vi "smith_analysis.vi"() -> ()   [LabVIEW 2013]
panel:
  out "appended array":dbl[][](array[numeric])=[[9086390000.0, 9086990000.0, 9087590000.0, 9088190000.0, 9088790000.0, 9089390000.0, 9089990000.0, 9090590000.0, 9091190000.0, 9091790000.0, 9092390000.0, 9092990000.0, 9093590000.0, 9094190000.0, 9094790000.0, 9095390000.0, 9095990000.0, 9096590000.0, 9097190000.0, 9097790000.0, 9098390000.0, 9098990000.0, 9099590000.0, 9100190000.0, 9100790000.0, 9101390000.0, 9101990000.0, 9102590000.0, 9103190000.0, 9103790000.0, 9104390000.0, 9104990000.0, 9105590000.0, 9106190000.0, 9106790000.0, 9107390000.0, 9107990000.0, 9108590000.0, 9109190000.0, 9109790000.0, 9110390000.0, 9110990000.0, 9111590000.0, 9112190000.0, 9112790000.0, 9113390000.0, 9113990000.0, 9114590000.0, 9115190000.0, 9115790000.0, 9116390000.0, 9116990000.0, 9117590000.0, 9118190000.0, 9118790000.0, 9119390000.0, 9119990000.0, 9120590000.0, 9121190000.0, 9121790000.0, 9122390000.0, 9122990000.0, 9123590000.0, 9124190000.0, 9124790000.0, 9125390000.0, 9125990000.0, 9126590000.0, 9127190000.0, 9127790000.0, 9128390000.0, 9128990000.0, 9129590000.0, 9130190000.0, 9130790000.0, 9131390000.0, 9131990000.0, 9132590000.0, 9133190000.0, 9133790000.0, 9134390000.0, 9134990000.0, 9135590000.0, 9136190000.0, 9136790000.0, 9137390000.0, 9137990000.0, 9138590000.0, 9139190000.0, 9139790000.0, 9140390000.0, 9140990000.0, 9141590000.0, 9142190000.0, 9142790000.0, 9143390000.0, 9143990000.0, 9144590000.0, 9145190000.0, 9145790000.0, 9146390000.0, 9146990000.0, 9147590000.0, 9148190000.0, 9148790000.0, 9149390000.0, 9149990000.0, 9150590000.0, 9151190000.0, 9151790000.0, 9152390000.0, 9152990000.0, 9153590000.0, 9154190000.0, 9154790000.0, 9155390000.0, 9155990000.0, 9156590000.0, 9157190000.0, 9157790000.0, 9158390000.0, 9158990000.0, 9159590000.0, 9160190000.0, 9160790000.0, 9161390000.0, 9161990000.0, 9162590000.0, 9163190000.0, 9163790000.0, 9164390000.0, 9164990000.0, 9165590000.0, 9166190000.0, 9166790000.0, 9167390000.0, 9167990000.0, 9168590000.0, 9169190000.0, 9169790000.0, 9170390000.0, 9170990000.0, 9171590000.0, 9172190000.0, 9172790000.0, 9173390000.0, 9173990000.0, 9174590000.0, 9175190000.0, 9175790000.0, 9176390000.0, 9176990000.0, 9177590000.0, 9178190000.0, 9178790000.0, 9179390000.0, 9179990000.0, 9180590000.0, 9181190000.0, 9181790000.0, 9182390000.0, 9182990000.0, 9183590000.0, 9184190000.0, 9184790000.0, 9185390000.0, 9185990000.0, 9186590000.0, 9187190000.0, 9187790000.0, 9188390000.0, 9188990000.0, 9189590000.0, 9190190000.0, 9190790000.0, 9191390000.0, 9191990000.0, 9192590000.0, 9193190000.0, 9193790000.0, 9194390000.0, 9194990000.0, 9195590000.0, 9196190000.0, 9196790000.0, 9197390000.0, 9197990000.0, 9198590000.0, 9199190000.0, 9199790000.0, 9200390000.0, 9200990000.0, 9201590000.0, 9202190000.0, 9202790000.0, 9203390000.0, 9203990000.0, 9204590000.0, 9205190000.0, 9205790000.0, 9206390000.0, 9206990000.0, 9207590000.0, 9208190000.0, 9208790000.0, 9209390000.0, 9209990000.0, 9210590000.0, 9211190000.0, 9211790000.0, 9212390000.0, 9212990000.0, 9213590000.0, 9214190000.0, 9214790000.0, 9215390000.0, 9215990000.0, 9216590000.0, 9217190000.0, 9217790000.0, 9218390000.0, 9218990000.0, 9219590000.0, 9220190000.0, 9220790000.0, 9221390000.0, 9221990000.0, 9222590000.0, 9223190000.0, 9223790000.0, 9224390000.0, 9224990000.0, 9225590000.0, 9226190000.0, 9226790000.0, 9227390000.0, 9227990000.0, 9228590000.0, 9229190000.0, 9229790000.0, 9230390000.0, 9230990000.0, 9231590000.0, 9232190000.0, 9232790000.0, 9233390000.0, 9233990000.0, 9234590000.0, 9235190000.0, 9235790000.0, 9236390000.0, 9236990000.0, 9237590000.0, 9238190000.0, 9238790000.0, 9239390000.0, 9239990000.0, 9240590000.0, 9241190000.0, 9241790000.0, 9242390000.0, 9242990000.0, 9243590000.0, 9244190000.0, 9244790000.0, 9245390000.0, 9245990000.0, 9246590000.0, 9247190000.0, 9247790000.0, 9248390000.0, 9248990000.0, 9249590000.0, 9250190000.0, 9250790000.0, 9251390000.0, 9251990000.0, 9252590000.0, 9253190000.0, 9253790000.0, 9254390000.0, 9254990000.0, 9255590000.0, 9256190000.0, 9256790000.0, 9257390000.0, 9257990000.0, 9258590000.0, 9259190000.0, 9259790000.0, 9260390000.0, 9260990000.0, 9261590000.0, 9262190000.0, 9262790000.0, 9263390000.0, 9263990000.0, 9264590000.0, 9265190000.0, 9265790000.0, 9266390000.0, 9266990000.0, 9267590000.0, 9268190000.0, 9268790000.0, 9269390000.0, 9269990000.0, 9270590000.0, 9271190000.0, 9271790000.0, 9272390000.0, 9272990000.0, 9273590000.0, 9274190000.0, 9274790000.0, 9275390000.0, 9275990000.0, 9276590000.0, 9277190000.0, 9277790000.0, 9278390000.0, 9278990000.0, 9279590000.0, 9280190000.0, 9280790000.0, 9281390000.0, 9281990000.0, 9282590000.0, 9283190000.0, 9283790000.0, 9284390000.0, 9284990000.0, 9285590000.0, 9286190000.0, 9286790000.0, 9287390000.0, 9287990000.0, 9288590000.0, 9289190000.0, 9289790000.0, 9290390000.0, 9290990000.0, 9291590000.0, 9292190000.0, 9292790000.0, 9293390000.0, 9293990000.0, 9294590000.0, 9295190000.0, 9295790000.0, 9296390000.0, 9296990000.0, 9297590000.0, 9298190000.0, 9298790000.0, 9299390000.0, 9299990000.0, 9300590000.0, 9301190000.0, 9301790000.0, 9302390000.0, 9302990000.0, 9303590000.0, 9304190000.0, 9304790000.0, 9305390000.0, 9305990000.0, 9306590000.0, 9307190000.0, 9307790000.0, 9308390000.0, 9308990000.0, 9309590000.0, 9310190000.0, 9310790000.0, 9311390000.0, 9311990000.0, 9312590000.0, 9313190000.0, 9313790000.0, 9314390000.0, 9314990000.0, 9315590000.0, 9316190000.0, 9316790000.0, 9317390000.0, 9317990000.0, 9318590000.0, 9319190000.0, 9319790000.0, 9320390000.0, 9320990000.0, 9321590000.0, 9322190000.0, 9322790000.0, 9323390000.0, 9323990000.0, 9324590000.0, 9325190000.0, 9325790000.0, 9326390000.0, 9326990000.0, 9327590000.0, 9328190000.0, 9328790000.0, 9329390000.0, 9329990000.0, 9330590000.0, 9331190000.0, 9331790000.0, 9332390000.0, 9332990000.0, 9333590000.0, 9334190000.0, 9334790000.0, 9335390000.0, 9335990000.0, 9336590000.0, 9337190000.0, 9337790000.0, 9338390000.0, 9338990000.0, 9339590000.0, 9340190000.0, 9340790000.0, 9341390000.0, 9341990000.0, 9342590000.0, 9343190000.0, 9343790000.0, 9344390000.0, 9344990000.0, 9345590000.0, 9346190000.0, 9346790000.0, 9347390000.0, 9347990000.0, 9348590000.0, 9349190000.0, 9349790000.0, 9350390000.0, 9350990000.0, 9351590000.0, 9352190000.0, 9352790000.0, 9353390000.0, 9353990000.0, 9354590000.0, 9355190000.0, 9355790000.0, 9356390000.0, 9356990000.0, 9357590000.0, 9358190000.0, 9358790000.0, 9359390000.0, 9359990000.0, 9360590000.0, 9361190000.0, 9361790000.0, 9362390000.0, 9362990000.0, 9363590000.0, 9364190000.0, 9364790000.0, 9365390000.0, 9365990000.0, 9366590000.0, 9367190000.0, 9367790000.0, 9368390000.0, 9368990000.0, 9369590000.0, 9370190000.0, 9370790000.0, 9371390000.0, 9371990000.0, 9372590000.0, 9373190000.0, 9373790000.0, 9374390000.0, 9374990000.0, 9375590000.0, 9376190000.0, 9376790000.0, 9377390000.0, 9377990000.0, 9378590000.0, 9379190000.0, 9379790000.0, 9380390000.0, 9380990000.0, 9381590000.0, 9382190000.0, 9382790000.0, 9383390000.0, 9383990000.0, 9384590000.0, 9385190000.0, 9385790000.0, 0.0], [1.0014470756472609, 0.9811749599727149, 0.975937039152533, 0.957404308515006, 0.9736018230093859, 0.9604604054761811, 0.9792049244201155, 1.0152541903970067, 1.004440422987172, 0.9669142300691471, 0.9778889586067279, 0.9827563524115415, 0.9889865842957853, 0.9705799067333685, 1.0100148361341221, 0.9773606743960654, 0.9646774483545443, 0.9704643155585843, 0.9783010544752769, 0.9951174837276988, 0.9574011288539037, 0.9859926147182249, 0.9669596436669335, 0.9920583106963926, 0.9854864109639495, 0.9799430549111374, 0.9769108482599617, 1.034057942667083, 0.9639858725088492, 0.9893429207880235, 0.9909416773256717, 0.9890686668064436, 0.983690008455327, 0.992837107143869, 0.9537054075489657, 1.0007092044221306, 0.9859170574219019, 0.9924581976110967, 0.9633179253367699, 0.9854993598276752, 0.9988614892860668, 1.004290542828067, 0.9951406919895751, 0.9595604473467628, 0.9755040689387509, 1.0066850706289576, 0.9666753740843728, 0.9797492943616066, 0.9891009789576483, 0.976218574351781, 0.9423483466974647, 0.9949809297127765, 0.9863441817937338, 0.9948322048119537, 0.981473364768583, 0.9999575553906259, 0.9933478773682365, 0.9952508245668754, 0.9823564820622492, 0.9847369655634216, 1.0210893363673963, 0.9954525985294357, 1.0004858497317275, 0.9660627936505503, 0.9850142439017647, 0.9689016818726742, 0.9772122398202737, 0.9773991677095369, 0.995057165612707, 0.9794999128822224, 0.9653556017088364, 0.9590793894023546, 0.9927546646176238, 0.973951113405735, 0.998351636736338, 0.97956788821144, 0.9539799170177218, 0.9835730149003353, 0.9872478691492744, 1.0022504649650081, 0.9943597265449575, 1.007315613095887, 1.016783886043785, 0.9699349529618666, 1.0102763892837336, 0.9819198699224674, 1.0011398706228367, 0.9854156883054559, 1.0057695829277393, 0.9742808082199741, 0.983537484305779, 0.9756139402394592, 0.9529997175528215, 0.9882672606378323, 0.9964646576378824, 1.0162769185869391, 0.9771113467798679, 0.9902362691931147, 0.9974945712236141, 0.9857676635027528, 0.990436808833684, 1.0100054750913074, 1.02277349272177, 0.9912131451821969, 0.9706813850121981, 0.9941292664957707, 0.9971653637847144, 0.9727308351939552, 0.9985557171670739, 0.990099281613391, 0.9592058080706113, 0.9850771730276339, 0.9579121848414565, 1.0413373602481122, 0.985479131778255, 0.9745571754831918, 0.9822577587259966, 1.0045577810317978, 0.9893107663949505, 0.979052992956135, 0.995395289845648, 1.003559463689938, 0.9627423299378147, 0.9818148736996156, 0.9911217507502924, 0.9691634713250117, 0.989465289500339, 0.9869127245666133, 1.0003808783369692, 0.9929945051626885, 1.0352322704115924, 0.9850581097960746, 0.9637516282967002, 0.9694897298412518, 0.9884441528397356, 0.995682923689632, 1.0029582140150322, 0.9816802190570769, 0.973562814550217, 0.9786970085879368, 1.0077631757583416, 0.9912918509414795, 0.9988234438690078, 0.9614578884461156, 0.9718322743908004, 0.9995513798844637, 1.0082429778200743, 1.0017536975084038, 1.0064115760126986, 0.9876507461851545, 0.956689385504372, 0.9661731716427335, 0.977175002325847, 0.9874001417065671, 0.9913195667202573, 1.0229947902987884, 0.9908230523450857, 0.9723595088037424, 1.0167086713851914, 1.0014221968876416, 0.9673383399753221, 0.9734357709886645, 0.9739288695081485, 0.9823171957631014, 0.9790041819946486, 0.9892116556181274, 0.9772477925686469, 1.0181758365556028, 1.001727376833795, 0.9683302069118086, 1.00198525147198, 0.9513182110513856, 0.9925278473984726, 0.9951607813898269, 0.9702746420708325, 0.9668003661435942, 0.9903244718945475, 1.0002563330224825, 0.9559761300224189, 0.974546529993097, 0.9995297116612798, 1.0046846903417743, 0.983485793116926, 1.0026831282008672, 0.9905199996322401, 0.9782269645034511, 1.0019674827158171, 0.9838323020512393, 0.9871369498901948, 1.0155032878430428, 1.0007802083671549, 0.9717739819680403, 0.9798965419234907, 0.9712219261120401, 0.9844985597447395, 0.9798576441835376, 0.9498016858038393, 0.9485857892398264, 0.9454073623982583, 1.0007271949801384, 0.9662435353148254, 0.9887495046962643, 0.9839744349092254, 0.9364946992801554, 0.9643564952803784, 0.9441374655249337, 0.971754009009434, 0.94475767751919, 0.9485826443001484, 0.9830282794482469, 0.9400594878438806, 0.9409738189508776, 0.9066711079610856, 0.915463647678557, 0.9396701651566188, 0.9520975581728508, 0.9423126541573191, 0.916329282360555, 0.921566191380927, 0.865778549512083, 0.8830002295417998, 0.9015180477343065, 0.8545954691171324, 0.8523334136356121, 0.8719727628977598, 0.8621363153292432, 0.8582191014270931, 0.8574731836182887, 0.8352852285636092, 0.8332663424689872, 0.8367676949759798, 0.8148731930380775, 0.768132593782985, 0.7554392738920802, 0.7742973748751909, 0.7692309771947555, 0.7361853856775491, 0.7229295395020657, 0.7162292618691556, 0.7153223511486996, 0.7038523932203432, 0.7046631520252984, 0.6876654171667271, 0.7131742885932114, 0.7295949009378736, 0.7202100019940961, 0.7169640294889787, 0.7255956374699953, 0.7200600365926345, 0.7328738917670794, 0.7451463019083417, 0.7501408073253467, 0.7860280564814197, 0.7502657987696241, 0.7949357397204114, 0.7308381467377276, 0.7339839462608265, 0.7818278743775611, 0.8228176839920871, 0.824930294322964, 0.7964975850050977, 0.851040653852145, 0.8674023224409153, 0.8329611929525236, 0.8653112375468961, 0.903797950771074, 0.904626553567601, 0.8942137089930287, 0.8929279570420267, 0.9161286665966389, 0.9213518446365686, 0.9337311542863986, 0.9132314115538239, 0.958929531207723, 0.9520449589749719, 0.9606968484432504, 0.9622764460410423, 0.9405015634503353, 0.9181830082029172, 0.9313713628937752, 0.9682831802106964, 0.9726380480876876, 0.9675825582307597, 0.9755855251096048, 0.9742205285306306, 0.938117519638244, 0.9894213001906471, 0.9623345999767065, 0.9579679485061534, 0.9742754606715178, 0.965359029778444, 0.9674215131103316, 0.999048768474733, 0.9660126446852795, 0.9718607497332871, 0.9884785831389925, 0.9889770052018733, 0.975942799652276, 0.9674709559003105, 0.9645214138379589, 0.9826473208551918, 0.9747900514559639, 1.0073417463170438, 0.9960191326890215, 0.9777628016062563, 0.9871572804153868, 0.979732602581617, 0.9621783501900804, 1.0035494562281797, 1.0234667718707915, 0.9744321465519066, 0.984978719422053, 0.9490304588181648, 0.960471232634771, 0.9586820282041454, 0.9952703809974975, 0.9935939138388714, 0.9798335301757216, 0.9818843448512631, 0.9981926711538844, 0.9667940944562141, 0.9930083650297539, 1.0042728940444805, 0.9833369795347292, 1.0017517424062143, 0.9753024253139055, 0.965200808574049, 0.9992128024341174, 0.9793024932726984, 1.0380638317887279, 1.00837436589276, 1.0087785666684708, 0.9932289237477132, 0.9881491713540708, 0.9823661949193174, 1.0071428430282414, 1.0047494405176227, 0.9697388231654123, 0.9955648663035147, 0.9757451117672439, 0.965899932555795, 0.995173946728936, 0.9733206750405338, 1.0100840183077469, 1.0205798795098242, 0.980784238323221, 0.9938809875634443, 0.9897960417826223, 0.9676963048194741, 0.9840107326075767, 0.9780538666413968, 0.989345322004715, 0.9725800113897322, 0.9962779298768482, 0.9932182218277528, 0.999048368598765, 0.997704205203082, 1.023055966550519, 0.9983091962952612, 1.0033860925619922, 1.001080262818101, 1.006336077516865, 0.9812156487589327, 0.9866191288790616, 0.9932778035890981, 0.9971510296100334, 0.9884139524995416, 0.9855924278511523, 1.000330267215062, 0.9864440374224626, 0.9988951742617913, 0.972420889326208, 0.9994224873830296, 0.9751213230562229, 1.0066958444054341, 1.0017026279702728, 1.006121603564702, 0.9998146288734505, 0.9982540880409198, 1.0006112606580864, 1.0132632628441745, 0.9930144225228087, 0.9855061019728004, 1.0075308285087101, 0.9923890673912591, 0.9971670909153905, 0.9717664358212392, 0.9955048167771158, 1.0050266914148576, 1.0040077203454065, 0.9901932888927553, 1.0091541117306855, 1.019794538829189, 0.9950871289946208, 1.0231463323788053, 1.0015788174867244, 1.0136704882172571, 1.0211076888102526, 0.9798691525864905, 0.9995206893815415, 0.9735533614336686, 1.002628630762015, 0.9994750433917784, 1.000155944068778, 1.017529542067576, 0.9799544605472695, 1.0316515030617535, 1.002642847473804, 1.0023056940563138, 1.0123473913122252, 0.9726947991595394, 1.005369366648692, 0.9840396822755659, 1.0056896524224046, 1.01572733967173, 1.0103478904427894, 0.9814616782229979, 0.9782889117845894, 1.014086059360066, 0.995592782365769, 0.9843930022872074, 0.981592310140594, 1.0063140840663636, 1.0314633136042046, 1.017532726011809, 0.9926552005635729, 0.9984222314433181, 1.0447708492117298, 0.9888363781653998, 0.9903881616210239, 1.007380501119788, 1.011313918741565, 0.9904087052704611, 0.9921574553892974, 0.9928362741761013, 0.9926441500650449, 1.0173265199849124, 1.0166826973787917, 1.0065300821749368, 1.01524847430923, 1.0070705109698126, 0.9961373671487929, 0.990351761612178, 0.9895118348580612, 1.0127139781004615, 0.9919064176994765, 1.028545864939614, 1.0056971745667131, 1.0083581919439726, 1.0124609854580402, 1.0136761439727657, 0.9840082996236655, 1.0202061013802584, 0.9984242505740754, 0.9879124268801043, 1.0037430715028068, 1.0192688458545662, 1.0271412752394748, 1.0166519570601582, 1.014684172103505, 0.9867195225358091, 1.0022951775500146, 1.0193250022609626, 1.0138811972269712, 1.0239886485911098, 0.9909066283639297, 1.0095574651413095, 1.0127093937926512, 0.9958766396951416, 1.002544645080407, 1.0168612717326622, 0.9920031388504779, 1.020492196904426, 1.0000446691737441, 0.9953733339559021, 0.9772444274510915, 0.9815990975221964, 1.0279212579067207, 1.00788685713182, 1.0201225100089373, 0.9909418829202061, 0.9974774481735453, 1.0001029038060412, 1.0100479902057737, 1.0105843722362406, 1.0246274087847818, 1.0087809391074272, 0.9827460582988843, 0.985266426382351, 1.0146552137268186, 1.018838611539896, 1.010283473938368, 1.0177839076299846, 1.0151865505681978, 1.000575066722015, 1.0201068151955661, 0.990512354022508, 1.0080336466892885, 1.0160074638707435, 0.9949843251549022, 1.0151315605240072]]
  in  "Path":path=path "/CCCP/Users/CCCP/creamy_seas/monday_starts_on_saturday/dipole/data_labview/4_smith/Qubit15_5JJ_1Jun05'17_smith_07"
  in  "SMOOTH N-points":i32=1
  in  "index 4":i32=2
  in  "length 3":i32=3
  in  "index 3":i32
  in  "Fit":bool
  out "Gamma1r (MHz)":dbl[](array[numeric])
  out "G1":dbl[][](array[numeric])=[[0.02022, 0.02022, 0.02022, 0.02022, 0.02022, 0.02022, 0.02022, 0.02022, 0.02022, 0.02022, 0.02022, 0.02022, 0.02022, 0.02022, 0.02022, 0.02022, 0.02022, 0.02022, 0.02022, 0.02022, 0.02022, 0.02022, 0.02022, 0.02022, 0.02022, 0.02022, 0.02022, 0.02022, 0.02022, 0.02022, 0.02022, 0.02022, 0.02022, 0.02022, 0.02022, 0.02022, 0.02022, 0.02022, 0.02022, 0.02022, 0.02022, 0.02022, 0.02022, 0.02022, 0.02022, 0.02022, 0.02022, 0.02022, 0.02022, 0.02022, 0.02022, 0.02022, 0.02022, 0.02022, 0.02022, 0.02022, 0.02022, 0.02022, 0.02022, 0.02022, 0.02022, 0.02022, 0.02022, 0.02022, 0.02022, 0.02022, 0.02022, 0.02022, 0.02022, 0.02022, 0.02022, 0.02022, 0.02022, 0.02022, 0.02022, 0.02022, 0.02022, 0.02022, 0.02022, 0.02022, 0.02022, 0.02022, 0.02022, 0.02022, 0.02022, 0.02022, 0.02022, 0.02022, 0.02022, 0.02022, 0.02022, 0.02022, 0.02022, 0.02022, 0.02022, 0.02022, 0.02022, 0.02022, 0.02022, 0.02022, 0.02022, 0.02022, 0.02022, 0.02022, 0.02022, 0.02022, 0.02022, 0.02022, 0.02022, 0.02022, 0.02022, 0.02022, 0.02022, 0.02022, 0.02022, 0.02022, 0.02022, 0.02022, 0.02022, 0.02022, 0.02022, 0.02022, 0.02022, 0.02022, 0.02022, 0.02022, 0.02022, 0.02022, 0.02022, 0.02022, 0.02022, 0.02022, 0.02022, 0.02022, 0.02022, 0.02022, 0.02022, 0.02022, 0.02022, 0.02022, 0.02022, 0.02022, 0.02022, 0.02022, 0.02022, 0.02022, 0.02022, 0.02022, 0.02022, 0.02022, 0.02022, 0.02022, 0.02022, 0.02022, 0.02022, 0.02022, 0.02022, 0.02022, 0.02022, 0.02022, 0.02022, 0.02022, 0.02022, 0.02022, 0.02022, 0.02022, 0.02022, 0.02022, 0.02022, 0.02022, 0.02022, 0.02022, 0.02022, 0.02022, 0.02022, 0.02022, 0.02022, 0.02022, 0.02022, 0.02022, 0.02022, 0.02022, 0.02022, 0.02022, 0.02022, 0.02022, 0.02022, 0.02022, 0.02022, 0.02022, 0.02022, 0.02022, 0.02022, 0.02022, 0.02022, 0.02022, 0.02022, 0.02022, 0.02022, 0.02022, 0.02022, 0.02022, 0.02022, 0.02022, 0.02022, 0.02022, 0.02022, 0.02022, 0.02022, 0.02022, 0.02022, 0.02022, 0.02022, 0.02022, 0.02022, 0.02022, 0.02022, 0.02022, 0.02022, 0.02022, 0.02022, 0.02022, 0.02022, 0.02022, 0.02022, 0.02022, 0.02022, 0.02022, 0.02022, 0.02022, 0.02022, 0.02022, 0.02022, 0.02022, 0.02022, 0.02022, 0.02022, 0.02022, 0.02022, 0.02022, 0.02022, 0.02022, 0.02022, 0.02022, 0.02022, 0.02022, 0.02022, 0.02022, 0.02022, 0.02022, 0.02022, 0.02022, 0.02022, 0.02022, 0.02022, 0.02022, 0.02022, 0.02022, 0.02022, 0.02022, 0.02022, 0.02022, 0.02022, 0.02022, 0.02022, 0.02022, 0.02022, 0.02022, 0.02022, 0.02022, 0.02022, 0.02022, 0.02022, 0.02022, 0.02022, 0.02022, 0.02022, 0.02022, 0.02022, 0.02022, 0.02022, 0.02022, 0.02022, 0.02022, 0.02022, 0.02022, 0.02022, 0.02022, 0.02022, 0.02022, 0.02022, 0.02022, 0.02022, 0.02022, 0.02022, 0.02022, 0.02022, 0.02022, 0.02022, 0.02022, 0.02022, 0.02022, 0.02022, 0.02022, 0.02022, 0.02022, 0.02022, 0.02022, 0.02022, 0.02022, 0.02022, 0.02022, 0.02022, 0.02022, 0.02022, 0.02022, 0.02022, 0.02022, 0.02022, 0.02022, 0.02022, 0.02022, 0.02022, 0.02022, 0.02022, 0.02022, 0.02022, 0.02022, 0.02022, 0.02022, 0.02022, 0.02022, 0.02022, 0.02022, 0.02022, 0.02022, 0.02022, 0.02022, 0.02022, 0.02022, 0.02022, 0.02022, 0.02022, 0.02022, 0.02022, 0.02022, 0.02022, 0.02022, 0.02022, 0.02022, 0.02022, 0.02022, 0.02022, 0.02022, 0.02022, 0.02022, 0.02022, 0.02022, 0.02022, 0.02022, 0.02022, 0.02022, 0.02022, 0.02022, 0.02022, 0.02022, 0.02022, 0.02022, 0.02022, 0.02022, 0.02022, 0.02022, 0.02022, 0.02022, 0.02022, 0.02022, 0.02022, 0.02022, 0.02022, 0.02022, 0.02022, 0.02022, 0.02022, 0.02022, 0.02022, 0.02022, 0.02022, 0.02022, 0.02022, 0.02022, 0.02022, 0.02022, 0.02022, 0.02022, 0.02022, 0.02022, 0.02022, 0.02022, 0.02022, 0.02022, 0.02022, 0.02022, 0.02022, 0.02022, 0.02022, 0.02022, 0.02022, 0.02022, 0.02022, 0.02022, 0.02022, 0.02022, 0.02022, 0.02022, 0.02022, 0.02022, 0.02022, 0.02022, 0.02022, 0.02022, 0.02022, 0.02022, 0.02022, 0.02022, 0.02022, 0.02022, 0.02022, 0.02022, 0.02022, 0.02022, 0.02022, 0.02022, 0.02022, 0.02022, 0.02022, 0.02022, 0.02022, 0.02022, 0.02022, 0.02022, 0.02022, 0.02022, 0.02022, 0.02022, 0.02022, 0.02022, 0.02022, 0.02022, 0.02022, 0.02022, 0.02022, 0.02022, 0.02022, 0.02022, 0.02022, 0.02022, 0.02022, 0.02022, 0.02022, 0.02022, 0.02022, 0.02022, 0.02022, 0.02022, 0.02022, 0.02022, 0.02022, 0.02022, 0.02022, 0.02022, 0.02022, 0.02022, 0.02022, 0.02022, 0.02022, 0.02022, 0.02022, 0.02022, 0.02022, 0.02022, 0.02022, 0.02022, 0.02022, 0.02022, 0.02022, 0.02022, 0.02022, 0.02022, 0.02022, 0.02022, 0.02022, 0.02022, 0.02022, 0.02022, 0.02022, 0.02022, 0.02022, 0.02022, 0.02022, 0.02022]]
  out "Manually fitted reflection 2":cluster{dbl[], "Array":dbl[]}[](graph)
  in  "G2":dbl=0.01011
  in  "x0 2":dbl=9.418
  in  "a 2":dbl=0.9
  in  "length":i32=1
  in  "index 2":i32=4
  out "Manually fitted reflection":cluster{dbl[], "Array":dbl[]}[](graph)
  in  "w":dbl=8e-05
  in  "a":dbl=0.55
  in  "x0":dbl=9.418
  in  "g1":dbl=0.02011
  out "Npowers":i16=8
  in  "length 2":i32=1
  out "Gamma2 (MHz)":dbl[](array[numeric])
  in  "index":i32=4
  out "a":dbl[][](array[numeric])
  in  "Points":u16=501
  in  "Span":dbl=300000000.0 format="%#_6p"
  in  "fc":dbl=9236390000.0 format="%#_6p"
  out "Extinction":cluster{dbl[], dbl[]}(graph)
  in  "r correnction":dbl=1.0
  out "fitted reflection":cluster{dbl[], "Array":dbl[]}[](graph)
  in  "Phase correction":dbl=-0.8200000000000005 step=0.01
  out "Smith":cluster{dbl[], dbl[]}[](graph)
  in  "String":string="CCCP:Users:CCCP:creamy_seas:monday_starts_on_saturday:dipole:data_labview:4_smith:Qubit15_5JJ_1Jun05'17_smith_22"
  out "Im(r)":cluster{dbl[], dbl[]}(graph)
  out "Re(r)":cluster{dbl[], dbl[]}(graph)
  # "Re[r]=a/(1+(2*(x-x0)/g)^2+2*(w/g)^2)\n\nassuming Gamma2=Gamma1/2"
  # "Re[r]=a/sqrt((1+((x-x0)/G2)*(x-x0)/G2))"
  # "Re[r]=a/(1+(2*(x-x0)/g)^2+2*(w/g)^2)\n\nassuming Gamma2=Gamma1/2"
  # "g2"
  # "x0"
  # "w"
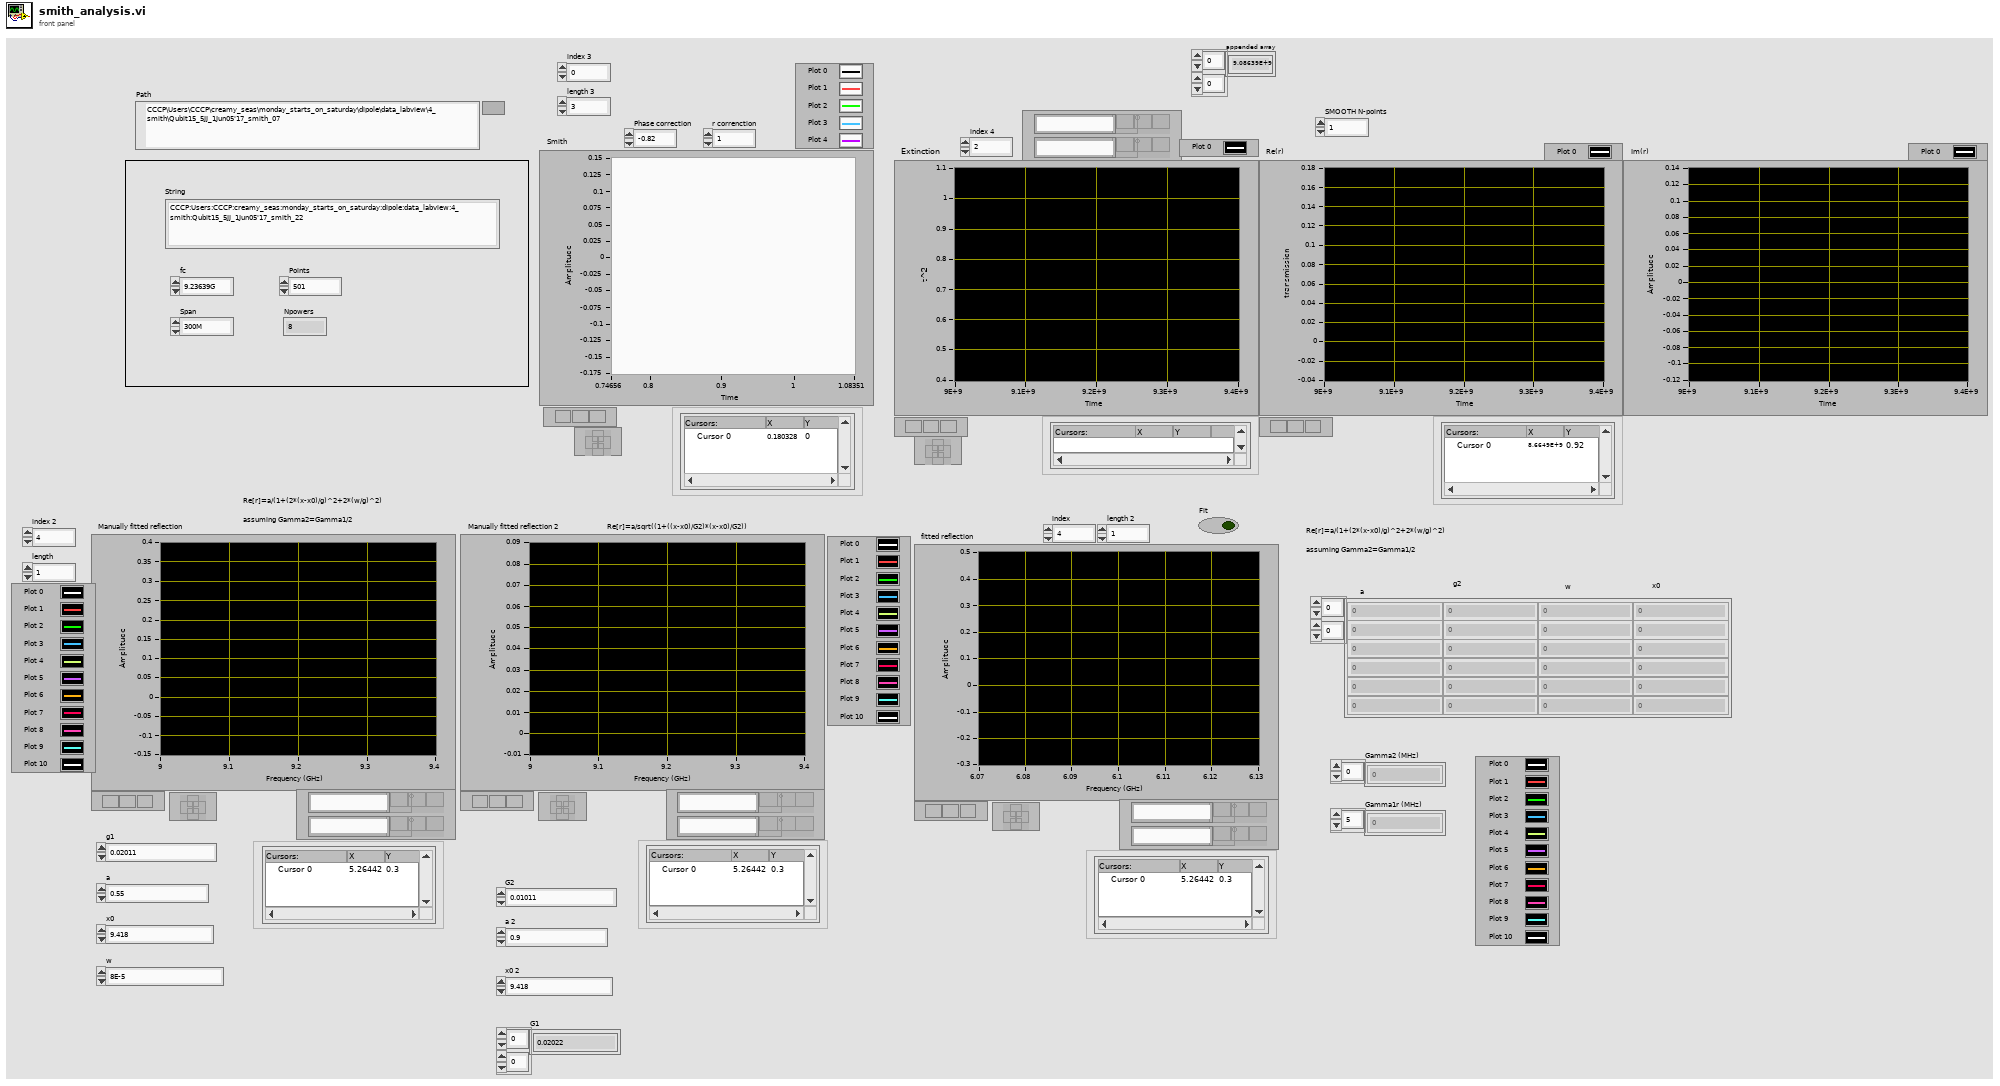
[diagram p1: front panel]
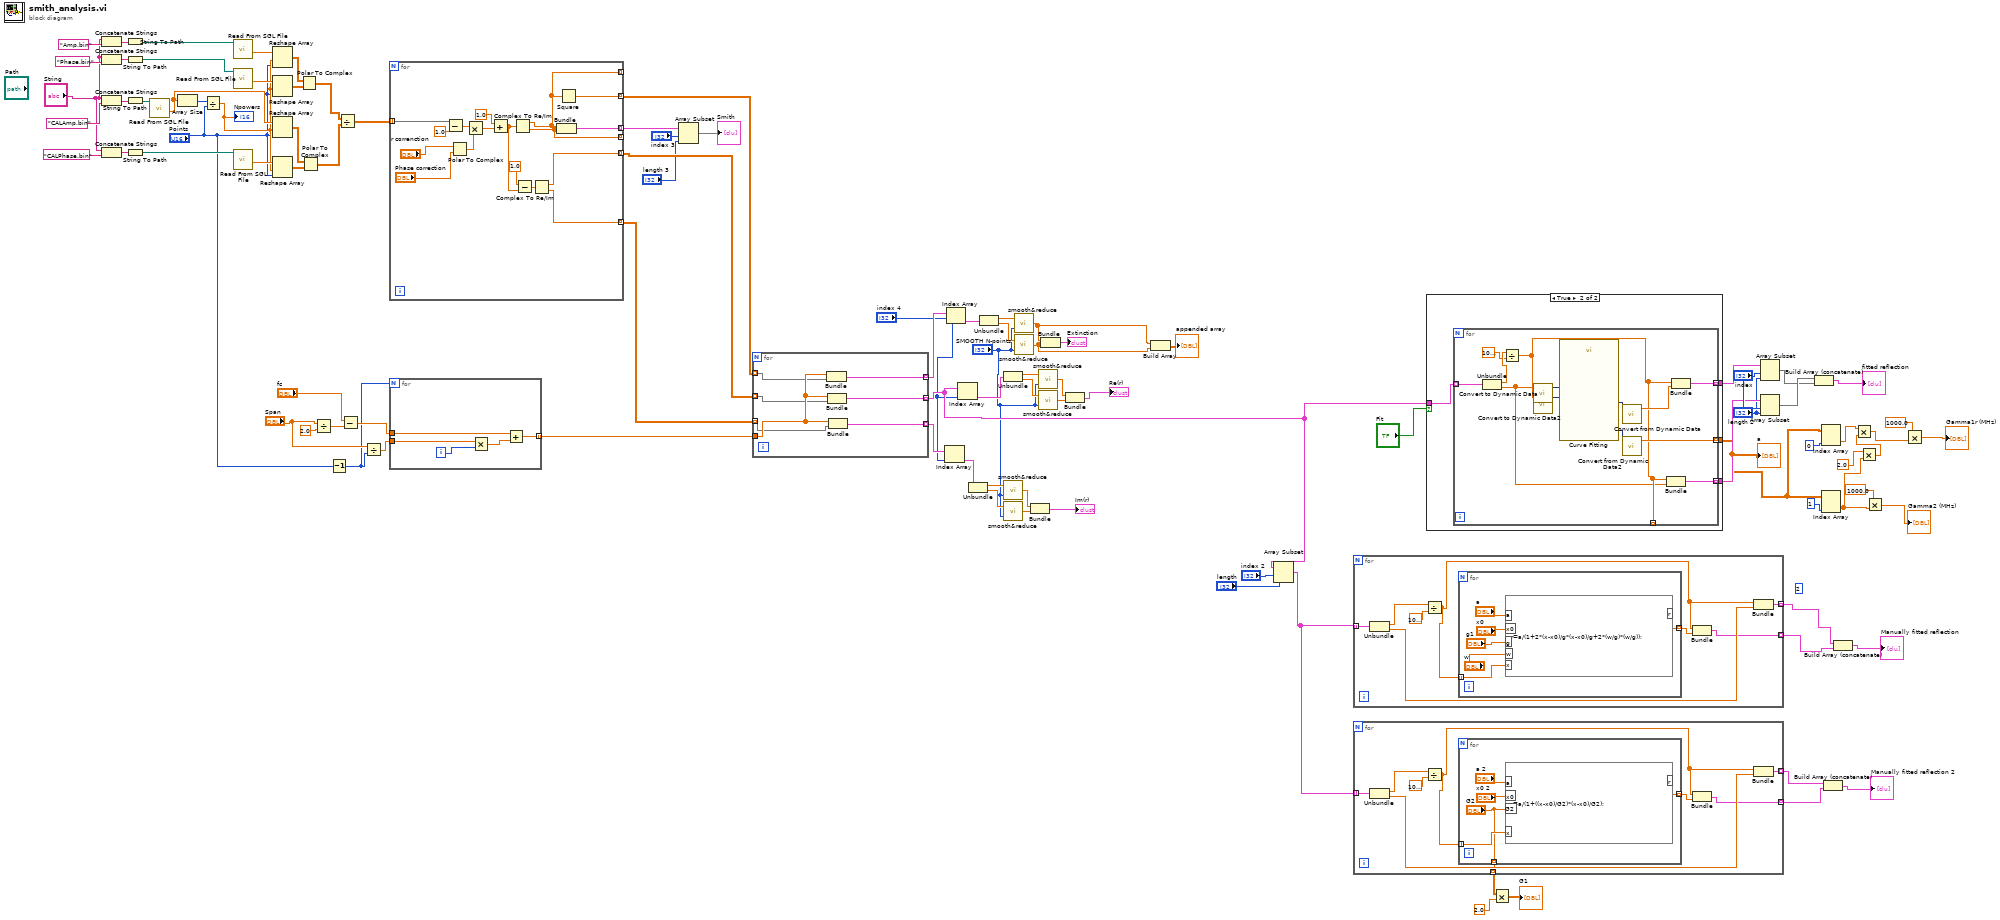
[diagram p0: block diagram]
diagram:
  (unwired) 2 ("index (row)")
  n1 = Concatenate Strings("String", "Amp.bin" ("File name")) -> (w75:string)
  n2 = Concatenate Strings("String", "Phase.bin" ("File name")) -> (w73:string)
  n3 = Concatenate Strings("String", "CALAmp.bin" ("File name")) -> (w79:string)
  n4 = Concatenate Strings("String", "CALPhase.bin" ("File name")) -> (w77:string)
  n5 = String To Path(string=w75) -> (path=w86:path)
  n6 = String To Path(string=w73) -> (path=w84:path)
  n7 = String To Path(string=w79) -> (path=w89:path)
  n8 = String To Path(string=w77) -> (path=w88:path)
  n9 = call <vilib>:"Read From SGL File.vi"("file path (dialog if empty)"=w89) -> ("1D array"=w72:sgl[])  [unwired: 6 in, 4 out]
  n10 = Array Size(array=w72) -> (size(s)=w70:i32)
  n11 = Divide(x=w70, y="Points") -> (x/y=w69:dbl)
  "Npowers" <- w69
  n12 = call <vilib>:"Read From SGL File.vi"("file path (dialog if empty)"=w86) -> ("1D array"=w85:sgl[])  [unwired: 6 in, 4 out]
  n13 = call <vilib>:"Read From SGL File.vi"("file path (dialog if empty)"=w84) -> ("1D array"=w83:sgl[])  [unwired: 6 in, 4 out]
  n14 = call <vilib>:"Read From SGL File.vi"("file path (dialog if empty)"=w88) -> ("1D array"=w87:sgl[])  [unwired: 6 in, 4 out]
  n15 = Reshape Array(w85, w69, "Points") -> (w68:sgl[][])
  n16 = Reshape Array(w83, w69, "Points") -> (w82:sgl[][])
  n17 = Reshape Array(w72, w69, "Points") -> (w71:sgl[][])
  n18 = Reshape Array(w87, w69, "Points") -> (w81:sgl[][])
  n19 = Polar To Complex(1:w82, 2:w68) -> (0:w66:csg[][])
  n20 = Polar To Complex(1:w81, 2:w71) -> (0:w65:csg[][])
  n21 = Divide(x="Span", y=2.0) -> (x/y=w61:dbl)
  n22 = Decrement(x="Points") -> (x-1=w51:u16)
  n23 = Divide(x=w66, y=w65) -> (x/y=w64:csg[][])
  n24 = Subtract(x="fc", y=w61) -> (x-y=w59:dbl)
  n25 = Divide(x="Span", y=w51) -> (x/y=w57:dbl)
  n26 = for {
    tunnel: w64 -> [w115] mode=indexing
    tunnel: [w107] -> w63 mode=indexing
    tunnel: [w106] -> w54 mode=indexing
    tunnel: [w101] -> w53 mode=indexing
    tunnel: [w102] -> w52 mode=indexing
    tunnel: [w100] -> _ mode=indexing
    tunnel: [w99] -> _ mode=indexing
    n27 = Subtract(x=w115, y=1.0 ("x")) -> (x-y=w113:cdb[])
    n28 = Polar To Complex(1:"Phase correction", 2:"r correnction") -> (0:w112:cdb)
    n29 = Multiply(x=w113, y=w112) -> (x*y=w109:cdb[])
    n30 = Add(x=1.0, y=w109) -> (x+y=w104:cdb[])
    n31 = Complex To Re/Im(x + iy=w104) -> (x=w100:dbl[], y=w99:dbl[])
    n32 = Subtract(x=1.0, y=w104) -> (x-y=w105:cdb[])
    n33 = Complex To Re/Im(x + iy=w105) -> (x=w101:dbl[], y=w102:dbl[])
    n34 = Bundle(w100, w99) -> (w107:cluster{dbl[], dbl[]})  [unwired: 1 in]
    n35 = Square(x=w100) -> (x^2=w106:dbl[])
  }
  n36 = for {
    N: w51 -> [_]
    tunnel: w59 -> [w118]
    tunnel: [w117] -> w55 mode=indexing
    tunnel: w57 -> [w116]
    i -> [w119]
    n37 = Multiply(x=w116, y=w119) -> (x*y=w120:dbl)
    n38 = Add(x=w118, y=w120) -> (x+y=w117:dbl)
  }
  n39 = Array Subset(array=w63, index="index 3", length="length 3") -> (→"Smith":cluster{dbl[], dbl[]}[])
  n40 = for {
    tunnel: w55 -> [w124]
    tunnel: w54 -> [w123] mode=indexing
    tunnel: w53 -> [w122] mode=indexing
    tunnel: w52 -> [w121] mode=indexing
    tunnel: [w127] -> w24 mode=indexing
    tunnel: [w126] -> w22 mode=indexing
    tunnel: [w125] -> w23 mode=indexing
    n41 = Bundle(w124, w123) -> (w127:cluster{dbl[], dbl[]})  [unwired: 1 in]
    n42 = Bundle(w124, w122) -> (w126:cluster{dbl[], dbl[]})  [unwired: 1 in]
    n43 = Bundle(w124, w121) -> (w125:cluster{dbl[], dbl[]})  [unwired: 1 in]
  }
  n44 = Index Array(array=w23, index="index 4") -> (element=w6:cluster{dbl[], dbl[]})
  n45 = Index Array(array=w24, index="index 4") -> (element=w20:cluster{dbl[], dbl[]})
  n46 = Index Array(array=w22, index="index 4") -> (element=w12:cluster{dbl[], dbl[]})
  n47 = Unbundle(w6) -> (w10:dbl[], w9:dbl[])
  n48 = Unbundle(w20) -> (w19:dbl[], w18:dbl[])
  n49 = Unbundle(w12) -> (w16:dbl[], w15:dbl[])
  n50 = call "smooth&reduce.vi"("N-points"="SMOOTH N-points", "Array in"=w10) -> ("Array out"=w8:dbl[])
  n51 = call "smooth&reduce.vi"("N-points"="SMOOTH N-points", "Array in"=w9) -> ("Array out"=w7:dbl[])
  n52 = call "smooth&reduce.vi"("N-points"="SMOOTH N-points", "Array in"=w19) -> ("Array out"=w3:dbl[])
  n53 = call "smooth&reduce.vi"("N-points"="SMOOTH N-points", "Array in"=w18) -> ("Array out"=w2:dbl[])
  n54 = Bundle("Array out"=w8, "Array out"=w7) -> (→"Im(r)":cluster{"Array out":dbl[], "Array out":dbl[]})  [unwired: 1 in]
  n55 = call "smooth&reduce.vi"("N-points"="SMOOTH N-points", "Array in"=w16) -> ("Array out"=w14:dbl[])
  n56 = call "smooth&reduce.vi"("N-points"="SMOOTH N-points", "Array in"=w15) -> ("Array out"=w13:dbl[])
  n57 = Bundle("Array out"=w3, "Array out"=w2) -> (→"Extinction":cluster{"Array out":dbl[], "Array out":dbl[]})  [unwired: 1 in]
  n58 = Bundle("Array out"=w14, "Array out"=w13) -> (→"Re(r)":cluster{"Array out":dbl[], "Array out":dbl[]})  [unwired: 1 in]
  n59 = Build Array(w3, w2) -> (→"appended array":dbl[][])
  n60 = Array Subset(array=w22, index="index 2", length="length") -> (w43:cluster{dbl[], dbl[]}[])
  n61 = for {
    tunnel: w43 -> [w135] mode=indexing
    tunnel: [w131] -> w46 mode=indexing
    tunnel: [w130] -> w49 mode=indexing
    n62 = Unbundle(w135) -> (w133:dbl[], w132:dbl[])
    n63 = Divide(x=w133, y=1000000000.0 ("x")) -> (x/y=w129:dbl[])
    n64 = for {
      tunnel: w129 -> [w137] mode=indexing
      tunnel: [w136] -> w128 mode=indexing
      n65 = formula code="r=a/(1+2*(x-x0)/g*(x-x0)/g+2*(w/g)*(w/g));"("a"="a", "x0"="x0", "g"="g1", "w"="w", "x"=w137) -> ("r"=w136:dbl)
    }
    n66 = Bundle(w129, w128) -> (w130:cluster{dbl[], dbl[]})  [unwired: 1 in]
    n67 = Bundle(w129, w132) -> (w131:cluster{dbl[], dbl[]})  [unwired: 1 in]
  }
  n68 = for {
    tunnel: w43 -> [w150] mode=indexing
    tunnel: [w146] -> w41 mode=indexing
    tunnel: [w145] -> w40 mode=indexing
    tunnel: [w142] -> w39 mode=indexing
    n69 = Unbundle(w150) -> (w148:dbl[], w147:dbl[])
    n70 = Divide(x=w148, y=1000000000.0 ("x")) -> (x/y=w144:dbl[])
    n71 = for {
      tunnel: w144 -> [w153] mode=indexing
      tunnel: [w152] -> w143 mode=indexing
      tunnel: ["G2"] -> w142 mode=indexing
      n72 = formula code="r=a/(1+((x-x0)/G2)*(x-x0)/G2);"("a"="a 2", "x0"="x0 2", "G2"="G2", "x"=w153) -> ("r"=w152:dbl)
    }
    n73 = Bundle(w144, w143) -> (w145:cluster{dbl[], dbl[]})  [unwired: 1 in]
    n74 = Bundle(w144, w147) -> (w146:cluster{dbl[], dbl[]})  [unwired: 1 in]
  }
  n75 = case shown="True" "Fit" {
    tunnel: [_ w159] -> w98
    tunnel: [_ w158] -> w93
    tunnel: [_ w157] -> w34
    tunnel: w22 -> [_ w156]
    frame False {
    }
    frame True {
      n76 = for {
        tunnel: w156 -> [w161] mode=indexing
        tunnel: [w168] -> w157 mode=indexing
        tunnel: [w166] -> w159 mode=indexing
        tunnel: [w165] -> w158 mode=indexing
        tunnel: [w162] -> _ mode=indexing
        n77 = Unbundle(w161) -> (w164:dbl[], w160:dbl[])
        n78 = Divide(x=w164, y=1000000000.0 ("x")) -> (x/y=w162:dbl[])
        n79 = call "Convert to Dynamic Data"("Array"=w160) -> ("Dynamic Data Type"=w169:dynamicdata)  [unwired: 3 in]
        n80 = call "Convert to Dynamic Data2"("Array"=w162) -> ("Dynamic Data Type"=w170:dynamicdata)  [unwired: 3 in]
        n81 = call "Curve Fitting"("Locations"=w170, "Signals"=w169) -> ("best fit"=w171:dynamicdata, "non-linear coefficients"=w172:dynamicdata)  [unwired: 5 in, 3 out]
        n82 = call "Convert from Dynamic Data"("Dynamic Data Type"=w171) -> ("Array"=w167:dbl[])  [unwired: 3 in]
        n83 = call "Convert from Dynamic Data2"("Dynamic Data Type"=w172) -> ("Array"=w168:dbl[])  [unwired: 3 in]
        n84 = Bundle(w162, w160) -> (w165:cluster{dbl[], dbl[]})  [unwired: 1 in]
        n85 = Bundle(w162, "Array"=w167) -> (w166:cluster{dbl[], "Array":dbl[]})  [unwired: 1 in]
      }
    }
  }
  "a" <- w34
  n86 = Multiply(x=w39, y=2.0 ("x")) -> (x*y=→"G1":dbl[][])
  n87 = Array Subset(array=w98, index="index", length="length 2") -> (w94:cluster{dbl[], "Array":dbl[]}[])
  n88 = Array Subset(array=w93, index="index", length="length 2") -> (w95:cluster{dbl[], dbl[]}[])
  n89 = Build Array (concatenate)(w95, w94) -> (→"fitted reflection":cluster{dbl[], "Array":dbl[]}[])
  n90 = Index Array(array=w34, index (col)=0 ("index (row)")) -> (element=w33:dbl[])  [unwired: 1 in]
  n91 = Index Array(array=w34, index (col)=1 ("index (row)")) -> (element=w31:dbl[])  [unwired: 1 in]
  n92 = Build Array (concatenate)(w41, w40) -> (→"Manually fitted reflection 2":cluster{dbl[], dbl[]}[])
  n93 = Build Array (concatenate)(w46, w49) -> (→"Manually fitted reflection":cluster{dbl[], dbl[]}[])
  n94 = Multiply(x=2.0, y=w31) -> (x*y=w30:dbl[])
  n95 = Multiply(x=w33, y=w30) -> (x*y=w28:dbl[])
  n96 = Multiply(x=1000.0, y=w31) -> (x*y=→"Gamma2 (MHz)":dbl[])
  n97 = Multiply(x=1000.0, y=w28) -> (x*y=→"Gamma1r (MHz)":dbl[])
